vi "Heat_Load_Calc_Red.vi"(8 "Input Array 2":dbl[](array[numeric]), 9 "Input Array":dbl[](array[numeric]), 10 "Avg Temp In":dbl, 11 "Temp In":dbl) -> (0 "Remaining Time Out (s)":dbl format="%.0g", 1 "Remaining Time Out":dbl format="%<%H:%M:%S>t", 2 "Output Array":dbl[](array[numeric]), 4 "% Complete":dbl)   [LabVIEW 2014]
panel:
  out "Ageing Time Out (s)":dbl format="%.0g"
  out "Ageing Time Out":dbl format="%<%H:%M:%S>t"
  in  "Ageing Time In":dbl
  out "k(i) Out":dbl
  in  "k(i) In":dbl
  # "Inputs"
  # "Outputs"
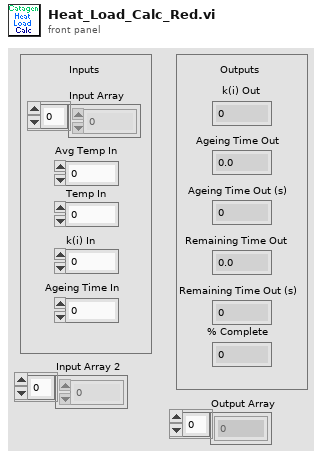
[diagram p1: front panel]
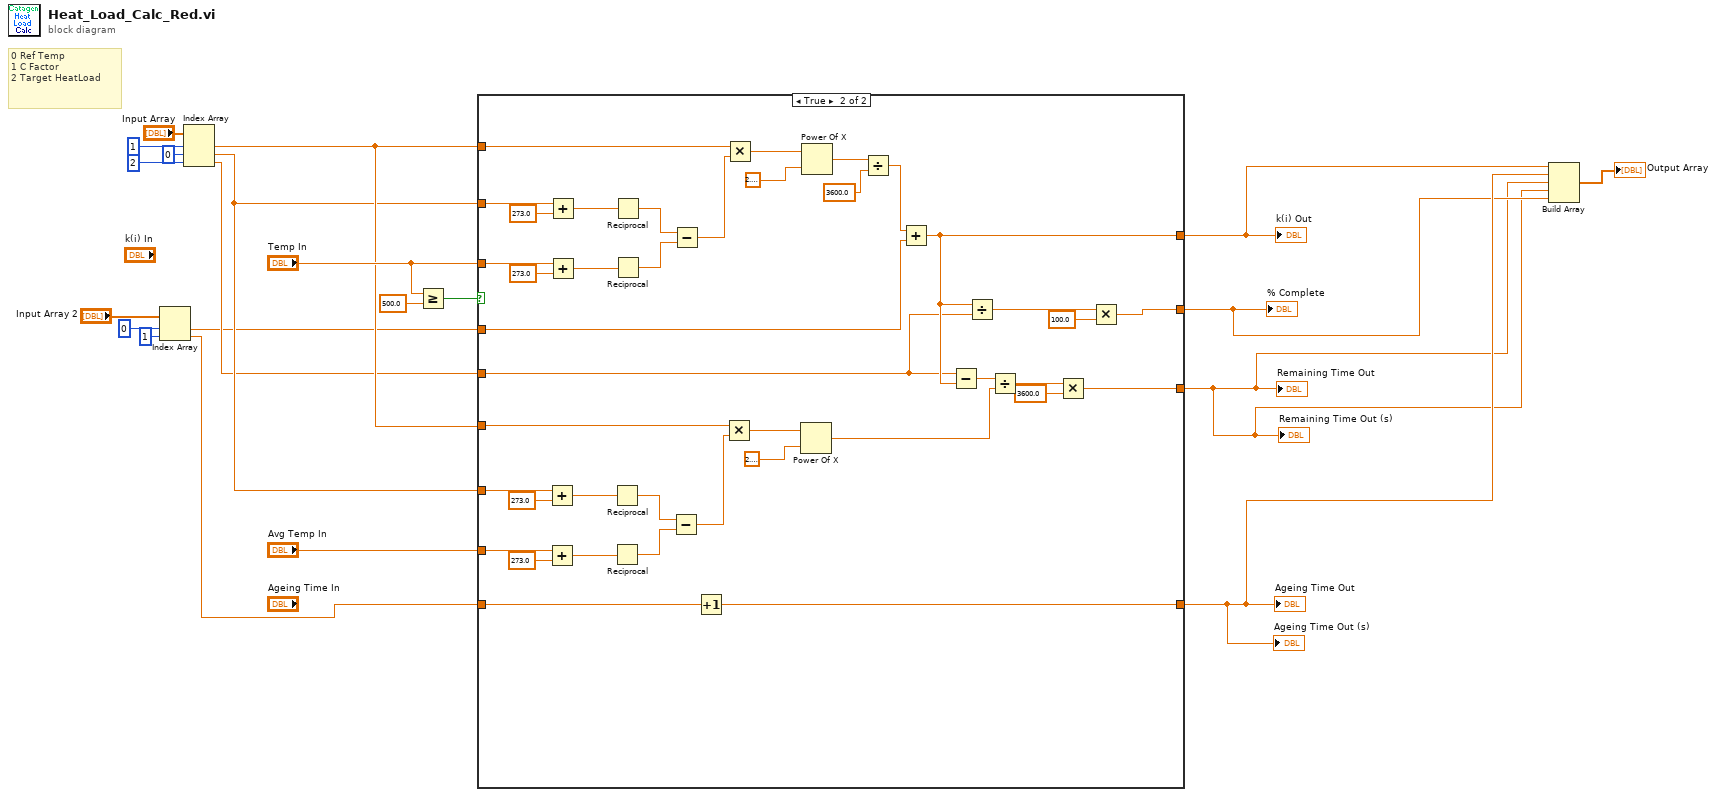
[diagram p0: block diagram]
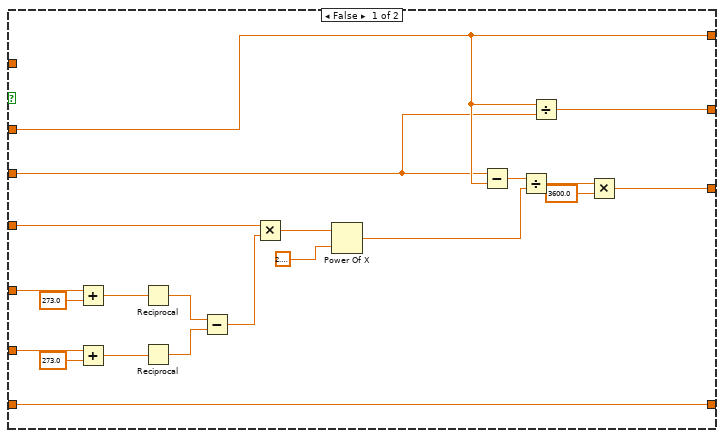
[diagram p2: hidden frame]
diagram:
  # "0 Ref Temp\n1 C Factor\n2 Target HeatLoad"
  n1 = Index Array(array="Input Array 2", index #1=0 ("index"), index #2=1 ("index")) -> (element #1=w5:dbl, element #2=w6:dbl)
  n2 = Index Array(array="Input Array", index #1=1 ("index"), index #2=0 ("index"), index #3=2 ("index")) -> (element #1=w17:dbl, element #2=w15:dbl, element #3=w14:dbl)
  n3 = Greater Or Equal?(x="Temp In", y=500.0) -> (x >= y?=w21:bool)
  n4 = case shown="True" w21 {
    tunnel: "Temp In" -> [_ w82]
    tunnel: w15 -> [_ w77]
    tunnel: w17 -> [_ w73]
    tunnel: w5 -> [w23 w70]
    tunnel: [w23 w44] -> w10
    tunnel: w6 -> [w42 w66]
    tunnel: [w42 w65] -> w9
    tunnel: w17 -> [w28 w55]
    tunnel: w15 -> [w27 w54]
    tunnel: "Avg Temp In" -> [w26 w53]
    tunnel: w14 -> [w22 w43]
    tunnel: [w25 w48] -> w1
    tunnel: [w24 w45] -> w2
    frame False {
      n5 = Add(x=w27, y=273.0) -> (x+y=w33:dbl)
      n6 = Add(x=w26, y=273.0) -> (x+y=w30:dbl)
      n7 = Reciprocal(x=w33) -> (1/x=w34:dbl)
      n8 = Reciprocal(x=w30) -> (1/x=w31:dbl)
      n9 = Subtract(x=w34, y=w31) -> (x-y=w35:dbl)
      n10 = Multiply(x=w28, y=w35) -> (x*y=w36:dbl)
      n11 = Power Of X(1:2.718281828459045, 2:w36) -> (0:w39:dbl)
      n12 = Subtract(x=w22, y=w23) -> (x-y=w38:dbl)
      n13 = Divide(x=w38, y=w39) -> (x/y=w40:dbl)
      n14 = Divide(x=w23, y=w22) -> (x/y=w24:dbl)
      n15 = Multiply(x=w40, y=3600.0) -> (x*y=w25:dbl)
    }
    frame True {
      n16 = Add(x=w54, y=273.0) -> (x+y=w60:dbl)
      n17 = Add(x=w53, y=273.0) -> (x+y=w63:dbl)
      n18 = Add(x=w77, y=273.0) -> (x+y=w76:dbl)
      n19 = Add(x=w82, y=273.0) -> (x+y=w80:dbl)
      n20 = Reciprocal(x=w60) -> (1/x=w59:dbl)
      n21 = Reciprocal(x=w63) -> (1/x=w62:dbl)
      n22 = Reciprocal(x=w76) -> (1/x=w75:dbl)
      n23 = Reciprocal(x=w80) -> (1/x=w79:dbl)
      n24 = Subtract(x=w59, y=w62) -> (x-y=w58:dbl)
      n25 = Subtract(x=w75, y=w79) -> (x-y=w74:dbl)
      n26 = Increment(x=w66) -> (x+1=w65:dbl)
      n27 = Multiply(x=w55, y=w58) -> (x*y=w57:dbl)
      n28 = Multiply(x=w73, y=w74) -> (x*y=w72:dbl)
      n29 = Power Of X(1:2.718281828459045, 2:w57) -> (0:w51:dbl)
      n30 = Power Of X(1:2.718281828459045, 2:w72) -> (0:w69:dbl)
      n31 = Divide(x=w69, y=3600.0) -> (x/y=w67:dbl)
      n32 = Add(x=w67, y=w70) -> (x+y=w44:dbl)
      n33 = Subtract(x=w43, y=w44) -> (x-y=w52:dbl)
      n34 = Divide(x=w44, y=w43) -> (x/y=w46:dbl)
      n35 = Divide(x=w52, y=w51) -> (x/y=w50:dbl)
      n36 = Multiply(x=w50, y=3600.0) -> (x*y=w48:dbl)
      n37 = Multiply(x=w46, y=100.0) -> (x*y=w45:dbl)
    }
  }
  "k(i) Out" <- w10
  "Ageing Time Out" <- w9
  "Ageing Time Out (s)" <- w9
  "Remaining Time Out" <- w1
  "Remaining Time Out (s)" <- w1
  "% Complete" <- w2
  n38 = Build Array(w10, w9, w1, w1, w2) -> (→"Output Array":dbl[])
